vi "Date_Time_Formater.vi"(1 "Date In":string="27-03-2020 10:09:07 AM") -> (0 "Date Out":timestamp)   [LabVIEW 2020]
panel:
  out "resulting string":string
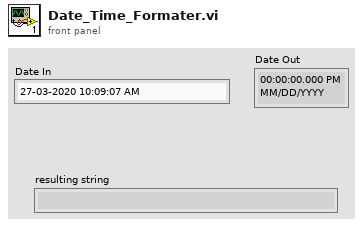
[diagram p1: front panel]
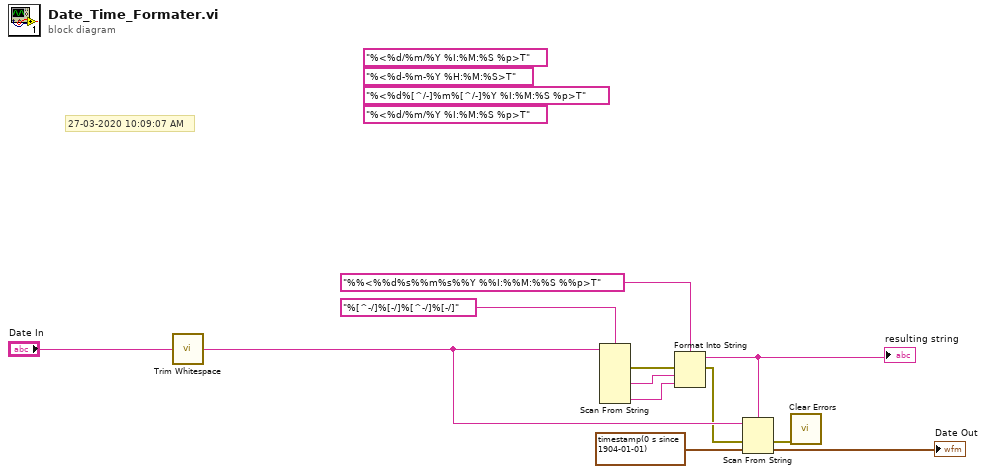
[diagram p0: block diagram]
diagram:
  (unwired) "%<%d/%m/%Y %I:%M:%S %p>T" ("time format string (%c)")
  (unwired) "%<%d/%m/%Y %I:%M:%S %p>T" ("time format string (%c)")
  (unwired) "%<%d-%m-%Y %H:%M:%S>T" ("time format string (%c)")
  (unwired) "%<%d%[^/-]%m%[^/-]%Y %I:%M:%S %p>T" ("time format string (%c)")
  # "27-03-2020 10:09:07 AM"
  n1 = call <vilib>:"Trim Whitespace.vi"("string"="Date In") -> ("trimmed string"=w6:string)  [unwired: 1 in]
  n2 = Scan From String(format string="%[^-/]%[-/]%[^-/]%[-/]", input string=w6) -> (error out=w3:errorcluster, output 2=w9:string, output 4=w8:string)  [unwired: 8 in, 2 out]
  n3 = Format Into String(format string="%%<%%d%s%%m%s%%Y %%I:%%M:%%S %%p>T" ("time format string (%c)"), error in=w3, w9, w8) -> (resulting string=w7:string, error out=w2:errorcluster)  [unwired: 1 in]
  "resulting string" <- w7
  n4 = Scan From String(format string=w7, input string=w6, error in=w2, default 1=timestamp(0 s since 1904-01-01) ("time stamp")) -> (error out=w1:errorcluster, output 1=→"Date Out":timestamp)  [unwired: 1 in, 2 out]
  n5 = call <vilib>:"Clear Errors.vi"("error in (no error)"=w1) -> ()  [unwired: 5 in, 2 out]
